vi "Dashboard Main.vi"() -> ()   [LabVIEW 2015]
uses:
  <vilib>/Utility/miscctls.llb/LVRowAndColumnTypeDef.ctl
  <vilib>/event_ctls.llb/eventvkey.ctl
  <vilib>/Rock Robotics/WPI/Dashboard/WPI_DashboardLogging Global.vi
  <vilib>/Rock Robotics/Network Tables/NT Read Numeric Array.vi
  <vilib>/Rock Robotics/Network Tables/SD Write Number.vi
  <vilib>/Rock Robotics/Network Tables/NT Write Boolean.vi
  <vilib>/Rock Robotics/Network Tables/NT Read Boolean.vi
  <vilib>/Utility/config.llb/Write Key (String).vi
  <vilib>/Utility/config.llb/Write Key (I32).vi
  <vilib>/Utility/config.llb/NI_LVConfig.lvlib
panel:
  in  "Vision 2":u16(ring)=3 items=["IP Camera"=3]
  out "Camera Image 2":T1(plugin-control)
  in  "TCP":refnum<k5>
  in  "Rec Mode":enum32{"Stop", "Record", "Playback"}(radio)
  in  "Vision":u16(ring)=1 items=["USB Cam"=1]
  out "Camera IP":string
  out "Image Message":string="Timeout in Camera Communications"
  in  "Dashboard Tab":T2(tab)
  in  "Camera Settings":T3={"Frame Rate"=30, "Compression"=30, "Size"=1} {"Frame Rate" scale=1.0..30.0; "Size" items=["640x480", "320x240", "160x120"]}
  out "Mode":T4(ring)=enum."Auto Disabled"
  in  "DB Camera Config":bool
  out "fps":dbl format="%#.1g"
  out "Mbps":dbl format="%#.1g"
  out "Mbps LED":bool
  in  "Autonomous Select":T5(ring)
  in  "Top Speed":dbl=1300.0 min=0.0 max=2.0 step=0.01
  in  "Intake Speed":dbl=1.0 min=0.0 max=1.0 step=0.01
  in  "Bottom Speed":dbl=2100.0 min=0.0 max=2.0 step=0.01
  in  "First  Drive":dbl=180.0 min=0.0 max=2.0 step=0.01
  in  "First Turn":dbl=39.0 min=0.0 max=1.0 step=0.01
  in  "Second Turn":dbl min=0.0 max=1.0 step=0.01
  in  "Second Drive":dbl=72.0 min=0.0 max=2.0 step=0.01
  in  "PID Control":bool=TRUE
  out "Bottom Encoder Velocity":dbl(knob) scale=0.0..3000.0
  out "Top Wop":bool
  out "Bottom Floop":bool
  out "Override":bool
  out "SHOOT!":bool
  in  "Auto Shoot":bool=TRUE
  in  "Release Speed":dbl=2090.0
  out "Line  Break":bool
  out "x":dbl
  out "y":dbl
  in  "Release Time":dbl=2090.0
  out "angle":dbl
  out "scale":dbl
  in  "DB/String 9":string
  in  "DB/String 8":string
  in  "DB/String 7":string
  in  "DB/String 6":string
  in  "DB/String 5":string
  in  "DB/String 4":string
  in  "DB/String 3":string
  in  "DB/String 2":string
  in  "DB/String 1":string
  in  "DB/String 0":string
  in  "DB/Slider 0":dbl(slide) scale=0.0..5.0
  in  "DB/Slider 1":dbl(slide) scale=0.0..5.0
  in  "DB/Slider 2":dbl(slide) scale=0.0..5.0
  in  "DB/Slider 3":dbl(slide) scale=0.0..5.0
  out "DB/LED 3":bool
  out "DB/LED 2":bool
  out "DB/LED 1":bool
  out "DB/LED 0":bool
  in  "DB/Button 3":bool
  in  "DB/Button 2":bool
  in  "DB/Button 1":bool
  in  "DB/Button 0":bool caption="New Name"
  out "Mbps 2":dbl format="%#.1g"
  in  "Camera Settings 2":T3={"Frame Rate"=30, "Compression"=30, "Size"=1} {"Frame Rate" scale=1.0..30.0; "Size" items=["640x480", "320x240", "160x120"]}
  out "fps 2":dbl format="%#.1g"
  in  "Rec Mode 2":enum32{"Stop", "Record", "Playback"}(radio)
  in  "Top P":dbl=3.0 min=0.0 max=2.0 step=0.01
  in  "Top I":dbl=0.01 min=0.0 max=1.0 step=0.01
  in  "Top D":dbl=7.0 min=0.0 max=2.0 step=0.01
  in  "Bottom P":dbl=3.0 min=0.0 max=2.0 step=0.01
  in  "Bottom I":dbl=0.01 min=0.0 max=1.0 step=0.01
  in  "Bottom D":dbl=12.0 min=0.0 max=2.0 step=0.01
  out "Gyro":dbl(knob) scale=0.0..360.0
  out "Top Encoder Velocity":dbl(knob) scale=0.0..3000.0
  in  "Gyro Reset":bool
  in  "Right Drive Reset":bool
  in  "Left Drive Reset":bool
  out "Left Drive Encoder":dbl
  out "Right Drive Encoder":dbl
  in  "X Offset":dbl min=0.0 max=1.0 step=0.01
  in  "Y Offset":dbl min=0.0 max=1.0 step=0.01
  in  "Angle Offset":dbl min=0.0 max=1.0 step=0.01
  in  "Scale Offset":dbl min=0.0 max=1.0 step=0.01
  in  "Test Slider":dbl(slide) scale=0.0..100.0 scale format="%#_3g"
  in  "On/Off":bool caption="Solenoid"
  in  "Test Name":u16(ring) items=["Select the test to run..."]
  in  "Test Tree":string(tree)
  in  "Motor":cluster{"Value":dbl, "Enable":bool} {"Value" scale=-1.0..1.0 scale format="%#_3g"}
  out "Progress":T6 {"Test Progress" scale=0.0..100.0}
  in  "Rev/Fwd":cluster{"Forward":bool, "Reverse":bool}
  in  "Test Ring":u16(ring) items=["Monochrome", "Color"]
  out "Cmd Status":string
  in  "Execute Command":bool
  in  "Command Params":string[][](table)
  in  "Command Selection":i32(listbox)
  in  "Select Auto":string(combo)
  out "JS2 Z":dbl(slide) scale=-1.0..1.0 scale format="%#_2e"
  out "JS2 Graph":cluster{"X":dbl, "Y":dbl}[](graph)
  out "JS2 Buttons":T7
  out "JS1 Z":dbl(slide) scale=-1.0..1.0 scale format="%#_2e"
  out "JS1 Graph":cluster{"X":dbl, "Y":dbl}[](graph)
  out "JS1 Buttons":T7
  in  "CheckList":i32(listbox)
  out "Tree":string(tree)
  out "Camera Image":T1(plugin-control)
  out "Background":bool
  # "This tab is a great place for autonomous settings and robot-specific values.\nPlace controls and indicators inside this tab and match name to\nDashboard Variables on robot. You can also delete this comment."
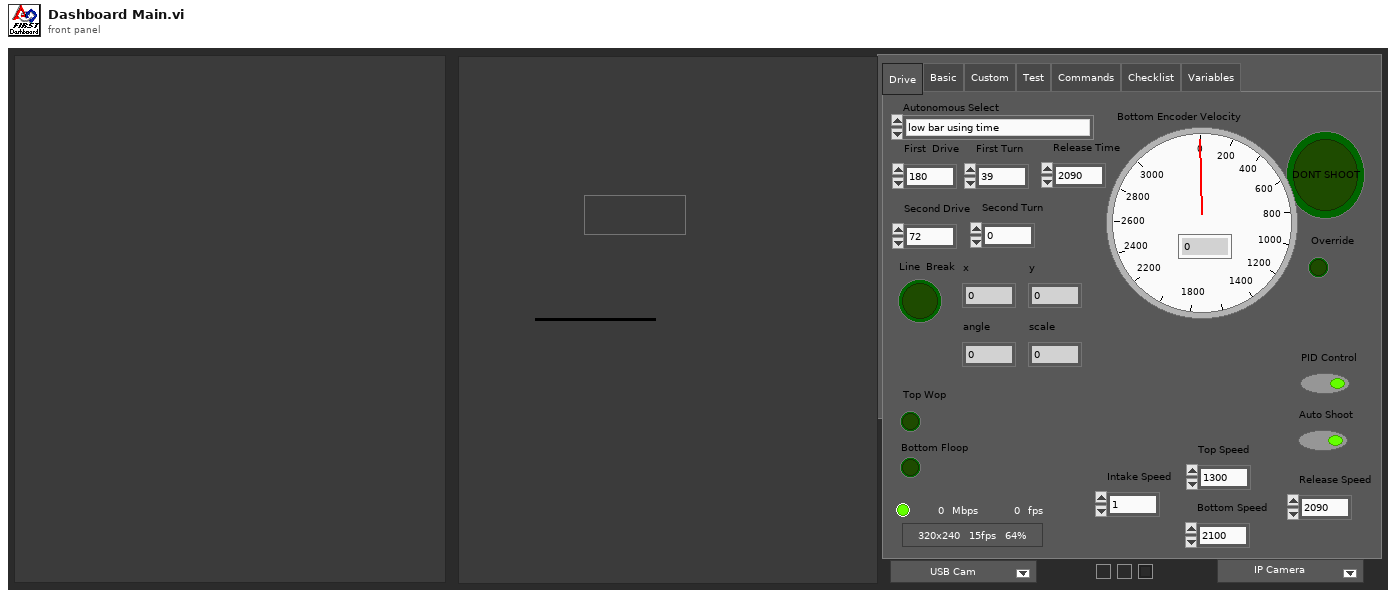
[diagram p1: front panel]
types:
  T1 = typedef "IMAQ Image.ctl" = refnum<image>
  T2 = enum32{"Drive", "Basic", "Custom", "Test", "Commands", "Checklist", "Variables"}
  T3 = cluster{"Frame Rate":i32, "Compression":i32, "Size":u16}
  T4 = enum8{"Tele-Op Disabled", "Tele-Op Enabled", "Auto Disabled", "Auto Enabled", "Test Disabled", "Test Enabled", "Disconnected", "No Code", "E-Stop"}
  T5 = enum16{"low bar using time", "low goal from low bar", "high goal from low bar", "rough terrain", "STRAIGHT FORWARD", "Do nothing", "low bar with encoder", "SHIMMY AUTO", "just touching", "Portcullis", "Cheval", "Vision 3rd Position", "Vision Test", "Bennett's Vision Code"}
  T6 = cluster{"Test Progress":u8, "Test Progress Text":string}
  T7 = cluster{bool, bool, bool, bool, bool, bool, bool, bool, bool, bool, bool, bool}
  T8 = typedef "Image Type" = u32
  T9 = cluster{"IDs":cluster{"RPC field ID":u16, "Unique ID":u16}, "String":string}
  T10 = enum32{"Drive", "Basic", "Custom", "Test", "Checklist", "Variables"}
  T11 = cluster{"Camera Image":refnum<vi>, "Dashboard Tab":refnum<vi>, "Background":refnum<vi>, "Vision":refnum<vi>, "Rec Mode":refnum<vi>, "Test Slider":refnum<vi>, "On/Off ":refnum<vi>, "Test Ring":refnum<vi>, "Rev/Fwd":refnum<vi>, "Test Name":refnum<vi>, "Motor":refnum<vi>, "Progress":refnum<vi>, "CheckList":refnum<vi>, "Tree":refnum<vi>, "Test Tree":refnum<vi>, "Command Params":refnum<vi>, "Command Selection":refnum<vi>, "Execute Command":refnum<vi>, "Cmd Status":refnum<vi>}
  T12 = cluster{"Position":cluster{"x":sgl, "y":sgl}, "Angle":sgl, "Scale":sgl, "Score":sgl, "Bounding Box":cluster{"x":sgl, "y":sgl}[]}[]
  T13 = cluster{"Position":cluster{"x":sgl, "y":sgl}, "Angle":sgl, "Scale":sgl, "Score":sgl, "Bounding Box":cluster{"x":sgl, "y":sgl}[]}
  T14 = typedef "NI_LVConfig.lvlib/Config Data RefNum.ctl" = refnum<k1>
  T15 = cluster{"Error Strings":string, "Disable Counts":cluster{u16, u16}, "Rail Faults":cluster{u16, u16, u16}, "Robot IP":string, "DB Mode":u8, "Event Info":cluster{"Name":string, "Type":u8, "Number":u16, "Replay":u8}, "Camera Addr":string}
  T16 = cluster{"Storage":cluster{"Disk Free":u64, "RAM Block":u32, "RAM free":u32}, "CPU Utilization":cluster{"CPU % ISR":sgl, "CPU % Time Crit":sgl, "CPU % Timed Str":sgl, "CPU % High":sgl, "CPU % Above":sgl, "CPU % Normal":sgl, "CPU % Low":sgl}, "CAN":cluster{"% Bus Utilization":sgl, "Bus Off Cnt":u32, "TX_FIFO Full Cnt":u32, "Receive Error Cnt":u8, "Transmit Error Cnt":u8}, "HID":cluster{"HID Outputs":u32, "Rumble Low":u16, "Rumble High":u16}[]}
  T17 = cluster{"Status bits":cluster{"Test Mode":bool, "Autonomous":bool, "Enabled":bool, "Code Start":bool, "Brownout":bool, "Reserved 2":bool, "Reserved 3":bool, "E-Stop":bool}, "Code Trace":cluster{"Disabled":bool, "TeleOp":bool, "Auto":bool, "Test":bool}, "Controller Type":enum16{"unknown", "cRIO", "roboRio"}, "Code?":enum16{"unknown", "noCode", "code"}, "Battery V":dbl}
  T18 = cluster{"Control Bits":cluster{"TestMode":bool, "Autonomous":bool, "Enabled":bool, "FMS Present":bool, bool, bool, bool, "E-Stop":bool}, "Team Station ":u8, "Countdown":sgl, "Joystick Values":cluster{"Axes":dbl[], "Buttons":bool[], "POVs":i16[]}[]}
  T19 = cluster{"Axes":dbl[], "Buttons":bool[], "POVs":i16[]}[]
  T20 = cluster{"Axes":dbl[], "Buttons":bool[], "POVs":i16[]}
  T21 = cluster{"Buttons[0]":bool, "Buttons[1]":bool, "Buttons[2]":bool, "Buttons[3]":bool, "Buttons[4]":bool, "Buttons[5]":bool, "Buttons[6]":bool, "Buttons[7]":bool, "Buttons[8]":bool, "Buttons[9]":bool, "Buttons[10]":bool, "Buttons[11]":bool}
  T22 = cluster{"Operation":enum16{"Update", "Clear"}, "Color Box":u32}[]
  T23 = typedef "eventvkey.ctl" = enum16{"ASCII", "Enter", "Return", "Shift", "Ctrl", "Alt", "Cmd", "Opt", "Caps", "NumLock", "Clear", "Break", "Up", "Down", "Left", "Right", "Insert", "Delete", "Home", "End", "PageUp", "PageDown", "Escape", "Help", "Pause", "ScrollLock", "F1", "F2", "F3", "F4", "F5", "F6", "F7", "F8", "F9", "F10", "F11", "F12", "F13", "F14", "F15", "F16", "F17", "F18", "F19", "F20", "F21", "F22", "F23", "F24", "Play", "VolumeUp", "VolumeDown", "Mute", "Two Byte Char"}
  T24 = cluster{"Image Size":bool, "Image Type":bool, "Pixel Value":bool, "ROI Information":bool, "Zoom Factor":bool}
  T25 = enum8{"Enabled", "Disabled", "Disabled and Grayed Out"}
  T26 = cluster{"Operation":enum16{"Update", "Clear"}, "Color Box":u32}
  T27 = typedef "LVRowAndColumnTypeDef.ctl" = cluster{"Row":i32, "Column":i32}
  T28 = cluster{"Shift":bool, "Ctrl":bool, "Alt":bool, "Cmd":bool, "Opt":bool}
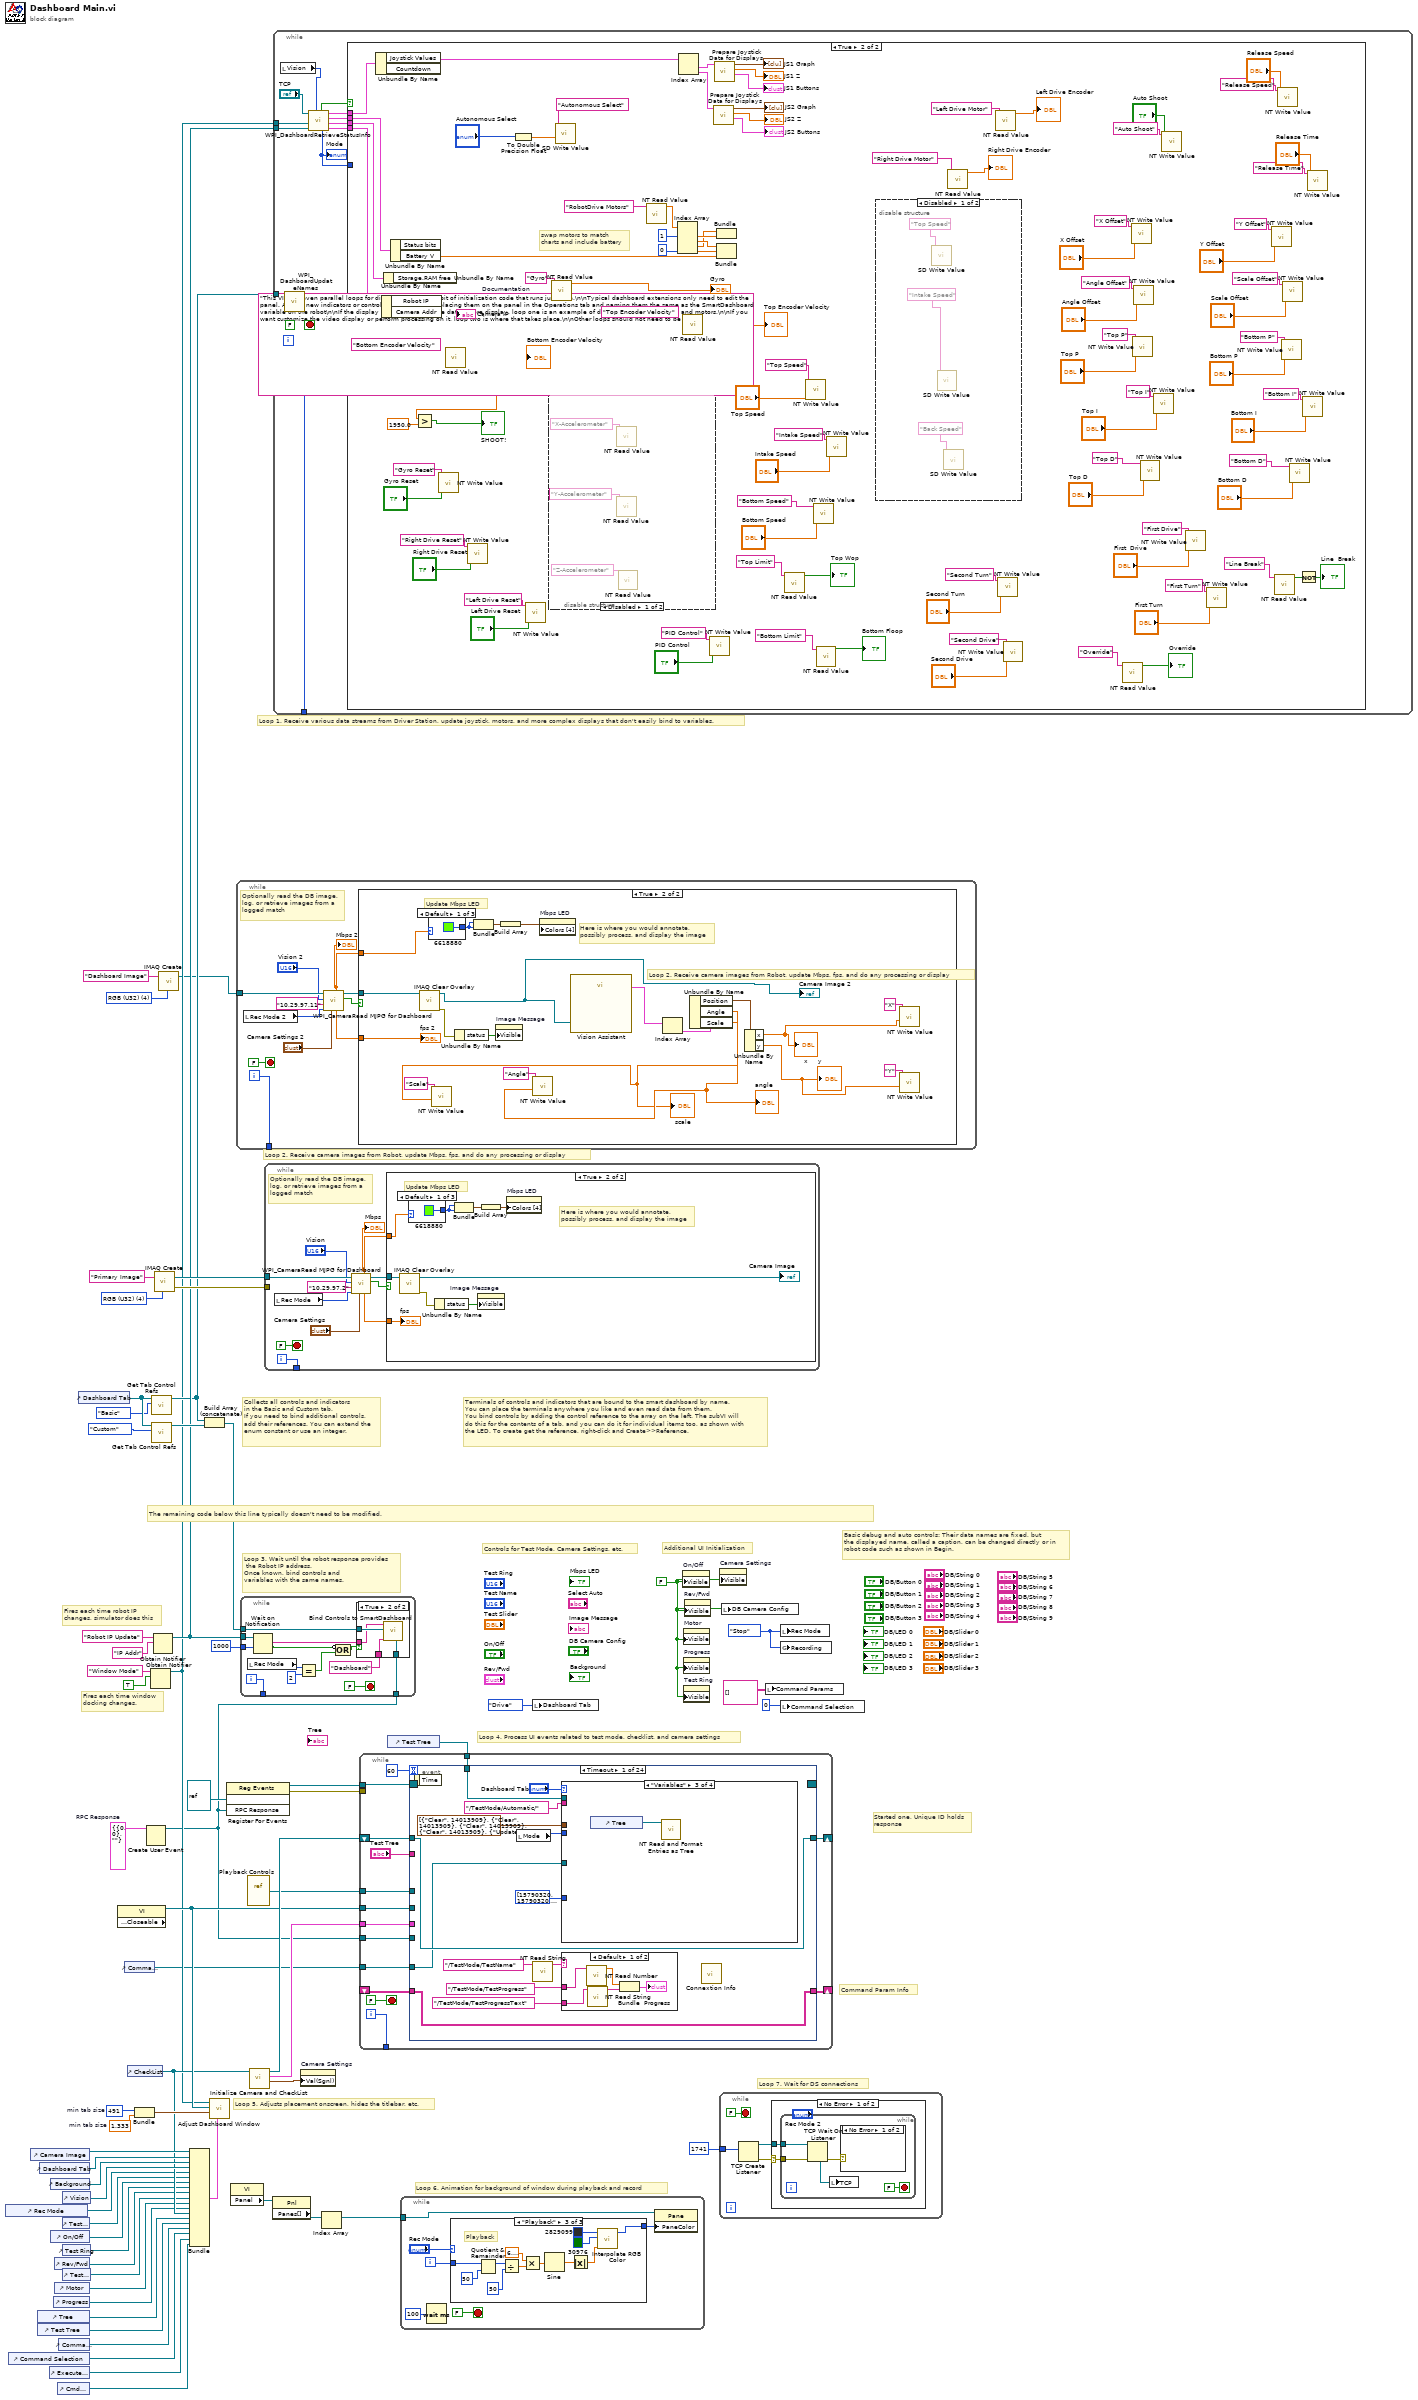
[diagram p0: block diagram]
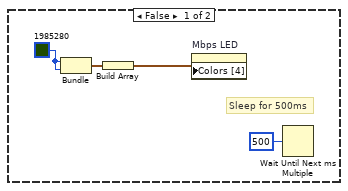
[diagram p2: hidden frame]
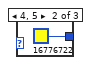
[diagram p3: hidden frame]
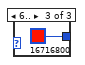
[diagram p4: hidden frame]
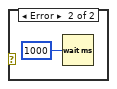
[diagram p5: hidden frame]
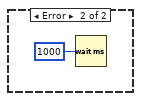
[diagram p6: hidden frame]
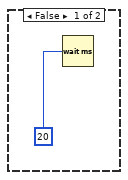
[diagram p7: hidden frame]
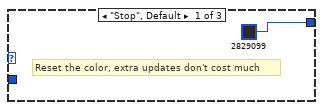
[diagram p10: hidden frame]
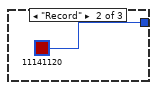
[diagram p11: hidden frame]
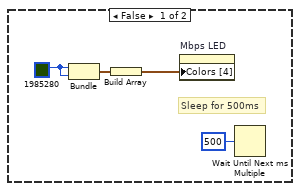
[diagram p13: hidden frame]
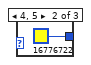
[diagram p14: hidden frame]
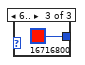
[diagram p15: hidden frame]
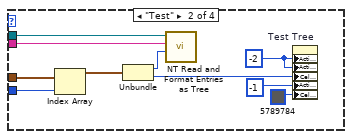
[diagram p17: hidden frame]
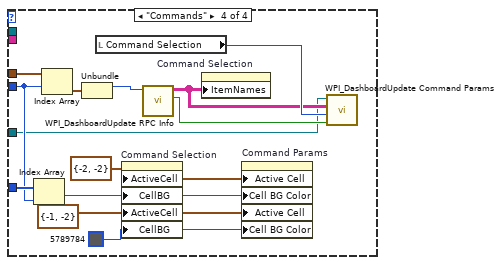
[diagram p18: hidden frame]
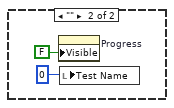
[diagram p19: hidden frame]
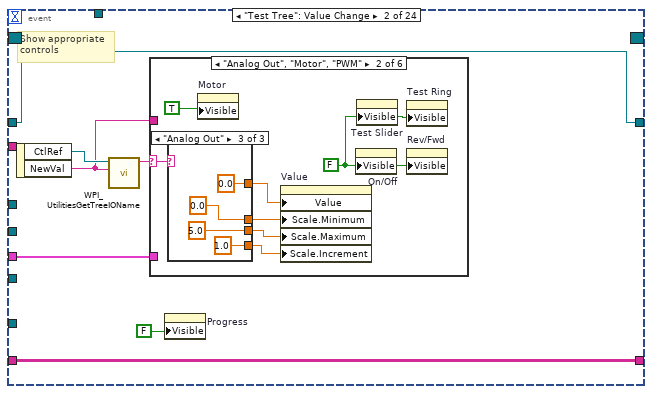
[diagram p20: hidden frame]
diagram:
  w2 = T8 4 items=["Grayscale (U8)", "Grayscale (I16)", "Grayscale (SGL)", "Complex (CSG)", "RGB (U32)", "HSL (U32)", "RGB (U64)"] ("Image Type")
  w10 = T9 {"IDs"={"RPC field ID"=0, "Unique ID"=0}, "String"=""}  # RPC Response
  w36 = 491  # min tab size
  w35 = 1.333  # min tab size
  w44 = enum32{"Stop", "Record", "Playback"}."Stop" ("Rec Mode")
  w18 = FALSE ("Visible")
  (unwired) "This VI has seven parallel loops for different tasks and a bit of initialization code that runs just once.\n\nTypical dashboard extensions only need to edit the panel. Adding new indicators or controls simply involves placing them on the panel in the Operations tab and naming them the same as the SmartDashboard variable on the robot\n\nIf the display needs to process the data before display, loop one is an example of doing that for the joysticks and motors.\n\nIf you want customize the video display or perform processing on it, loop two is where that takes place.\n\nOther loops should not need to be modified. They are pretty standard, and document the task they perform."  # Documentation
  w64 = T8 4 items=["Grayscale (U8)", "Grayscale (I16)", "Grayscale (SGL)", "Complex (CSG)", "RGB (U32)", "HSL (U32)", "RGB (U64)"] ("Image Type")
  # "Loop 2. Receive camera images from Robot, update Mbps, fps, and do any processing or display"
  # "Command Param Info"
  # "Started one, Unique ID holds\nresponse"
  # "Loop 7. Wait for DS connections"
  # "Basic debug and auto controls: Their data names are fixed, but\nthe displayed name, called a caption, can be changed directly or in\nrobot code such as shown in Begin."
  # "Controls for Test Mode, Camera Settings, etc."
  # "Additional UI Initialization"
  # "Loop 6. Animation for background of window during playback and record"
  # "Fires each time robot IP\nchanges, simulator does this"
  # "Fires each time window\ndocking changes."
  # "Collects all controls and indicators\nin the Basic and Custom tab.\nIf you need to bind additional controls,\nadd their references. You can extend the\nenum constant or use an integer."
  # "The remaining code below this line typically doesn't need to be modified."
  # "Loop 4. Process UI events related to test mode, checklist, and camera settings"
  # "Terminals of controls and indicators that are bound to the smart dashboard by name.\nYou can place the terminals anywhere you like and even read data from them.\nYou bind controls by adding the control reference to the array on the left. The subVI will\ndo this for the contents of a tab, and you can do it for individual items too, as shown with\nthe LED. To create get the reference, right-click and Create>>Reference."
  # "Loop 3. Wait until the robot response provides\n the Robot IP address.\nOnce known, bind controls and\nvariables with the same names."
  # "Loop 5. Adjusts placement onscreen, hides the titlebar, etc."
  # "Loop 1. Receive various data streams from Driver Station, update joystick, motors, and more complex displays that don't easily bind to variables."
  # "Loop 2. Receive camera images from Robot, update Mbps, fps, and do any processing or display"
  n1 = control-ref of="Rec Mode"() -> (w24:refnum<vi>)
  n2 = control-ref of="Command Selection"() -> (w9:refnum<vi>)
  n3 = control-ref of="Camera Image"() -> (w39:refnum<vi>)
  n4 = control-ref of="Tree"() -> (w28:refnum<vi>)
  n5 = control-ref of="Test Tree"() -> (w27:refnum<vi>)
  n6 = control-ref of="Dashboard Tab"() -> (w38:refnum<vi>)
  n7 = control-ref of="Execute Command"() -> (w11:refnum<vi>)
  n8 = control-ref of="Background"() -> (w33:refnum<vi>)
  n9 = control-ref of="On/Off"() -> (w22:refnum<vi>)
  n10 = control-ref of="Progress"() -> (w19:refnum<vi>)
  n11 = control-ref of="Rev/Fwd"() -> (w20:refnum<vi>)
  n12 = control-ref of="Motor"() -> (w25:refnum<vi>)
  n13 = control-ref of="Cmd Status"() -> (w5:refnum<vi>)
  n14 = control-ref of="Command Params"() -> (w12:refnum<vi>)
  n15 = control-ref of="Test Slider"() -> (w23:refnum<vi>)
  n16 = control-ref of="Vision"() -> (w37:refnum<vi>)
  n17 = control-ref of="Test Ring"() -> (w21:refnum<vi>)
  n18 = control-ref of="Test Name"() -> (w26:refnum<vi>)
  n19 = control-ref of="Dashboard Tab"() -> (w42:refnum<vi>)
  n20 = property class="VI" props=["Front Panel.Closeable"]() -> (reference out=w43:refnum<vi>)  [unwired: 2 in, 2 out]
  n21 = control-ref of="Command Params"() -> (w4:refnum<vi>)
  n22 = control-ref of="CheckList"() -> (w29:refnum<vi>)
  n23 = Bundle("min tab size"=w36, "min tab size"=w35) -> (w34:cluster{"min tab size":i32, "min tab size":dbl})  [unwired: 1 in]
  n24 = Create User Event(user event datatype=w10) -> (user event=w6:refnum<user-event>)  [unwired: 1 in, 1 out]
  n25 = Obtain Notifier(name (unnamed)="Window Mode", notification data type=TRUE) -> (notifier out=w15:refnum<notifier>)  [unwired: 2 in, 2 out]
  n26 = call <vilib>:"Get Tab Control Refs.vi"("Page Index"=T10."Basic" ("Dashboard Tab"), "TabControl in"=w42) -> ("ControlsOnPage"=w16:refnum<vi>[])  [unwired: 9 in]
  n27 = call <vilib>:"Get Tab Control Refs.vi"("Page Index"=T10."Custom" ("Dashboard Tab"), "TabControl in"=w42) -> ("ControlsOnPage"=w41:refnum<vi>[])  [unwired: 9 in]
  n28 = Obtain Notifier(name (unnamed)="Robot IP Update", notification data type="IP Addr" ("name (unnamed)")) -> (notifier out=w17:refnum<notifier>)  [unwired: 2 in, 2 out]
  n29 = call "IMAQ Create"("Image Name"="Primary Image", "Image Type"=w64) -> ("New Image"=w62:T1, "error out"=w61:errorcluster)  [unwired: 2 in, 1 out]
  n30 = call "IMAQ Create"("Image Name"="Dashboard Image", "Image Type"=w2) -> ("New Image"=w1:T1)  [unwired: 2 in, 2 out]
  n31 = Bundle("Camera Image"=w39, "Dashboard Tab"=w38, "Background"=w33, "Vision"=w37, "Rec Mode"=w24, "Test Slider"=w23, "On/Off"=w22, "Test Ring"=w21, "Rev/Fwd"=w20, "Test Name"=w26, "Motor"=w25, "Progress"=w19, "CheckList"=w29, "Tree"=w28, "Test Tree"=w27, "Command Params"=w12, "Command Selection"=w9, "Execute Command"=w11, "Cmd Status"=w5) -> (w30:T11)  [unwired: 1 in]
  n32 = Build Array (concatenate)(w16, w41) -> (w40:refnum<vi>[])
  n33 = call "Adjust Dashboard Window.vi"("Sizing Refnums"=w30, "Size Constraints"=w34, "VI"=w43, "WIn Mode"=w15) -> ()  [unwired: 8 in]
  n34 = register-events(refnum<vi> refnum, w6) -> (reference out=w48:refnum<event-registration>, error out=w47:errorcluster)  [unwired: 2 in]
  n35 = property class="VI"() -> ("Panel"=w51:refnum<vi>)  [unwired: 2 in, 2 out]
  n36 = while {
    tunnel: w1 -> [w73]
    tunnel: [w74] -> _
    i -> [w74]
    stop <- FALSE stop-if-true
    # "Optionally read the DB image,\nlog, or retrieve images from a\nlogged match"
    n37 = local read "Rec Mode 2"() -> (w68:enum32{"Stop", "Record", "Playback"})
    n38 = call <vilib>:"WPI_CameraRead MJPG for Dashboard.vi"("Camera Settings"="Camera Settings 2", "Rec Mode"=w68, "Camera IP"="10.29.97.11", "Camera Mode"="Vision 2", "Refnum in"=w73) -> ("Active"=w71:bool, "Refnum out"=w72:T1, "FPS"=w70:dbl, "Bandwidth (Mbps)"=w66:dbl)  [unwired: 3 in]
    "Mbps 2" <- w66
    n39 = case shown="True" w71 {
      tunnel: w72 -> [_ w96]
      tunnel: w66 -> [_ w95]
      tunnel: w70 -> [_ w94]
      frame False {
        w77 = u32 1985280 ("Color Box")
        # "Sleep for 500ms"
        n40 = Bundle("Color Box"=w77, "Color Box"=w77) -> (w78:cluster{"Color Box":u32, "Color Box":u32})  [unwired: 1 out]
        n41 = Build Array(w78) -> (w76:cluster{"Color Box":u32, "Color Box":u32}[])
        n42 = property on="Mbps LED" class="Bool (strict)"("Colors [4]"=w76) -> ()  [unwired: 2 in, 2 out]
        n43 = Wait Until Next ms Multiple(millisecond multiple=u32 500) -> ()  [unwired: 1 out]
      }
      frame True {
        # "Here is where you would annotate,\npossibly process, and display the image"
        # "Update Mbps LED"
        n44 = call "IMAQ Clear Overlay"("Image"=w96) -> ("error out"=w99:errorcluster, "Image Out"=w80:T1)  [unwired: 2 in, 7 out]
        "Camera Image 2" <- w80
        n45 = case shown="Default" w95 {
          tunnel: [u32 6618880 ("Color Box") u32 16776722 ("Color Box") u32 16716800 ("Color Box")] -> w97
          frame Default {
          }
          frame 4, 5 {
          }
          frame 6.. {
          }
        }
        n46 = Unbundle By Name(w99) -> ("status"=w92:bool)
        n47 = Bundle("Color Box"=w97, "Color Box"=w97) -> (w98:cluster{"Color Box":u32, "Color Box":u32})  [unwired: 1 out]
        n48 = property on="Image Message" class="Str"("Visible"=w92) -> ()  [unwired: 2 in, 2 out]
        n49 = Build Array(w98) -> (w93:cluster{"Color Box":u32, "Color Box":u32}[])
        n50 = property on="Mbps LED" class="Bool (strict)"("Colors [4]"=w93) -> ()  [unwired: 2 in, 2 out]
        n51 = call "Vision Assistant"("Image In"=w80) -> ("Calibrated Matches (Pattern Matching 1)"=w89:T12)  [unwired: 22 in, 4 out]
        n52 = Index Array(array=w89) -> (element=w91:T13)  [unwired: 1 in]
        n53 = Unbundle By Name(w91) -> ("Position"=w90:cluster{"x":sgl, "y":sgl}, "Angle"=w82:sgl, "Scale"=w81:sgl)
        "angle" <- w82
        "scale" <- w81
        n54 = call-poly <vilib>:"NT Write Value.vi"("Numeric"=w81, "Name"="Scale") -> ()  [unwired: 9 in, 1 out]
        n55 = call-poly <vilib>:"NT Write Value.vi"("Numeric"=w82, "Name"="Angle") -> ()  [unwired: 9 in, 1 out]
        n56 = Unbundle By Name(w90) -> ("x"=w87:sgl, "y"=w85:sgl)
        "x" <- w87
        "y" <- w85
        n57 = call-poly <vilib>:"NT Write Value.vi"("Numeric"=w87, "Name"="X") -> ()  [unwired: 9 in, 1 out]
        n58 = call-poly <vilib>:"NT Write Value.vi"("Numeric"=w85, "Name"="Y") -> ()  [unwired: 9 in, 1 out]
        "fps 2" <- w94
      }
    }
  }
  n59 = while {
    tunnel: w40 -> [w115]
    tunnel: w17 -> [w113]
    tunnel: [w111] -> _
    tunnel: u32 1000 ("milliseconds to wait") -> [w110]
    tunnel: w6 -> [w103]
    i -> [w111]
    stop <- FALSE stop-if-true
    n60 = local read "Rec Mode"() -> (w106:enum32{"Stop", "Record", "Playback"})
    n61 = Wait on Notification(notifier=w113, timeout in ms (-1)=w110) -> (notification=w112:string, timed out?=w108:bool)  [unwired: 2 in, 2 out]
    n62 = Equal?(x=w106, y=u16 2 ("Rec Mode")) -> (x = y?=w107:bool)
    n63 = Compound Arithmetic op=OR(invert w108, w107) -> (w109:bool)
    n64 = case shown="True" w109 {
      tunnel: w115 -> [_ w119]
      tunnel: w112 -> [_ w118]
      tunnel: "Dashboard" -> [_ w117]
      tunnel: w103 -> [_ w116]
      frame False {
      }
      frame True {
        n65 = call <vilib>:"Bind Controls to SmartDashboard.vi"("RPC ref"=w116, "Client Name"=w117, "Bound Control Refs"=w119, "Server IP Address"=w118) -> ()  [unwired: 8 in]
      }
    }
  }
  n66 = vi-ref "Playback Controls.vi"() -> (w49:refnum<vi>)
  n67 = call "Initialize Camera and CheckList.vi"("ListBox in"=w29) -> ("Cluster"=w55:cluster{"value":i32, "value":i32, "index":i32}, "Array"=w56:cluster{string[]}[], "File Refnum"=w54:T14)  [unwired: 8 in]
  n68 = while {
    tunnel: w62 -> [w128]
    tunnel: w61 -> [_]
    tunnel: [w129] -> _
    i -> [w129]
    stop <- FALSE stop-if-true
    # "Optionally read the DB image,\nlog, or retrieve images from a\nlogged match"
    n69 = local read "Rec Mode"() -> (w123:enum32{"Stop", "Record", "Playback"})
    n70 = call <vilib>:"WPI_CameraRead MJPG for Dashboard.vi"("Camera Settings"="Camera Settings", "Rec Mode"=w123, "Camera IP"="10.29.97.2", "Camera Mode"="Vision", "Refnum in"=w128) -> ("Active"=w126:bool, "Refnum out"=w127:T1, "FPS"=w125:dbl, "Bandwidth (Mbps)"=w121:dbl)  [unwired: 3 in]
    "Mbps" <- w121
    n71 = case shown="True" w126 {
      tunnel: w127 -> [_ w138]
      tunnel: w121 -> [_ w137]
      tunnel: w125 -> [_ w135]
      frame False {
        w131 = u32 1985280 ("Color Box")
        # "Sleep for 500ms"
        n72 = Bundle("Color Box"=w131, "Color Box"=w131) -> (w133:cluster{"Color Box":u32, "Color Box":u32})  [unwired: 1 out]
        n73 = Build Array(w133) -> (w132:cluster{"Color Box":u32, "Color Box":u32}[])
        n74 = property on="Mbps LED" class="Bool (strict)"("Colors [4]"=w132) -> ()  [unwired: 2 in, 2 out]
        n75 = Wait Until Next ms Multiple(millisecond multiple=u32 500) -> ()  [unwired: 1 out]
      }
      frame True {
        # "Here is where you would annotate,\npossibly process, and display the image"
        # "Update Mbps LED"
        n76 = call "IMAQ Clear Overlay"("Image"=w138) -> ("error out"=w142:errorcluster, "Image Out"=→"Camera Image":T1)  [unwired: 2 in, 7 out]
        n77 = case shown="Default" w137 {
          tunnel: [u32 6618880 ("Color Box") u32 16776722 ("Color Box") u32 16716800 ("Color Box")] -> w139
          frame Default {
          }
          frame 4, 5 {
          }
          frame 6.. {
          }
        }
        n78 = Unbundle By Name(w142) -> ("status"=w143:bool)
        n79 = Bundle("Color Box"=w139, "Color Box"=w139) -> (w141:cluster{"Color Box":u32, "Color Box":u32})  [unwired: 1 out]
        n80 = property on="Image Message" class="Str"("Visible"=w143) -> ()  [unwired: 2 in, 2 out]
        n81 = Build Array(w141) -> (w140:cluster{"Color Box":u32, "Color Box":u32}[])
        n82 = property on="Mbps LED" class="Bool (strict)"("Colors [4]"=w140) -> ()  [unwired: 2 in, 2 out]
        "fps" <- w135
      }
    }
  }
  n83 = property class="Pnl"(reference=w51) -> ("Panes[]"=w52:refnum<vi>[])  [unwired: 1 in, 2 out]
  n84 = while {
    tunnel: [w158] -> _
    tunnel: w17 -> [w152]
    tunnel: w16 -> [w151]
    tunnel: w15 -> [w147]
    i -> [w158]
    stop <- FALSE stop-if-true
    n85 = local read "Vision"() -> (w149:u16)
    n86 = call <vilib>:"WPI_DashboardUpdateNames.vi"("Controls on Tab"=w151) -> ()  [unwired: 11 in]
    n87 = call <vilib>:"WPI_DashboardRetrieveStatusInfo.vi"("Vision"=w149, "Binding Refnum"=w152, "Window Mode Notifier"=w147, "TCP Cnx"="TCP") -> ("Power and Errors"=w153:T15, "Robot Metrics"=w156:T16, "Status Info"=w157:T17, "Control Info"=w154:T18, "Robot Mode"=w150:T4, "Process?"=w155:bool)  [unwired: 2 in]
    "Mode" <- w150
    n88 = case shown="True" w155 {
      tunnel: w157 -> [_ w255]
      tunnel: w156 -> [_ w254]
      tunnel: w154 -> [_ w253]
      tunnel: w153 -> [_ w252]
      tunnel: w150 -> [_ _]
      frame False {
        n89 = Wait (ms)(milliseconds to wait=u32 20) -> ()  [unwired: 1 out]
      }
      frame True {
        # "swap motors to match\ncharts and include battery"
        n90 = Unbundle By Name(w253) -> ("Joystick Values"=w244:T19)  [unwired: 1 out]
        n91 = Unbundle By Name(w252) -> ("Camera Addr"=→"Camera IP":string)  [unwired: 1 out]
        n92 = Unbundle By Name(w254) -> ()  [unwired: 1 out]
        n93 = Unbundle By Name(w255) -> ("Battery V"=w245:dbl)  [unwired: 1 out]
        n94 = call-poly <vilib>:"NT Write Value.vi"("Boolean"="Gyro Reset", "Name"="Gyro Reset") -> ()  [unwired: 9 in, 1 out]
        n95 = call-poly <vilib>:"NT Read Value.vi"("Name"="Bottom Encoder Velocity") -> ("Numeric"=w175:dbl)  [unwired: 9 in, 1 out]
        "Bottom Encoder Velocity" <- w175
        n96 = Greater?(x=w175, y=1950.0) -> (0:→"SHOOT!":bool)
        n97 = call-poly <vilib>:"NT Write Value.vi"("Boolean"="Right Drive Reset", "Name"="Right Drive Reset") -> ()  [unwired: 9 in, 1 out]
        n98 = To Double Precision Float(number="Autonomous Select") -> (double precision float=w230:dbl)
        n99 = call-poly <vilib>:"NT Write Value.vi"("Boolean"="Left Drive Reset", "Name"="Left Drive Reset") -> ()  [unwired: 9 in, 1 out]
        n100 = disable-structure shown="Disabled" {
          frame Disabled {
            n101 = call-poly <vilib>:"NT Read Value.vi"("Name"="Y-Accelerometer") -> ("Numeric"=w266:dbl)  [unwired: 9 in, 1 out]
            n102 = call-poly <vilib>:"NT Read Value.vi"("Name"="X-Accelerometer") -> ("Numeric"=w265:dbl)  [unwired: 9 in, 1 out]
            n103 = call-poly <vilib>:"NT Read Value.vi"("Name"="Z-Accelerometer") -> ("Numeric"=w263:dbl)  [unwired: 9 in, 1 out]
          }
          frame Enabled {
          }
        }
        n104 = call-poly <vilib>:"NT Read Value.vi"("Name"="Gyro") -> ("Numeric"=→"Gyro":dbl)  [unwired: 9 in, 1 out]
        n105 = call-poly <vilib>:"SD Write Value.vi"("Numeric"=w230, "Name"="Autonomous Select") -> ()  [unwired: 8 in, 2 out]
        n106 = call-poly <vilib>:"NT Read Value.vi"("Name"="RobotDrive Motors") -> ("Numeric Array"=w233:dbl[])  [unwired: 9 in, 1 out]
        n107 = Index Array(array=w233, index #1=1, index #4=0) -> (element #1=w247:dbl, element #2=w248:dbl, element #3=w246:dbl, element #4=w251:dbl)  [unwired: 2 in]
        n108 = Index Array(array=w244) -> (element #1=w243:T20, element #2=w238:T20)  [unwired: 2 in]
        n109 = call-poly <vilib>:"NT Read Value.vi"("Name"="Top Encoder Velocity") -> ("Numeric"=→"Top Encoder Velocity":dbl)  [unwired: 9 in, 1 out]
        n110 = call-poly <vilib>:"NT Write Value.vi"("Boolean"="PID Control", "Name"="PID Control") -> ()  [unwired: 9 in, 1 out]
        n111 = call "Prepare Joystick Data for Displays.vi"("Joystick Values"=w238) -> ("Buttons"=→"JS2 Buttons":T21, "Z Axis"=→"JS2 Z":dbl, "Cartesian Data"=→"JS2 Graph":cluster{"X axis":dbl, "X axis":dbl}[])  [unwired: 8 in]
        n112 = call "Prepare Joystick Data for Displays.vi"("Joystick Values"=w243) -> ("Buttons"=→"JS1 Buttons":T21, "Z Axis"=→"JS1 Z":dbl, "Cartesian Data"=→"JS1 Graph":cluster{"X axis":dbl, "X axis":dbl}[])  [unwired: 8 in]
        n113 = Bundle("Numeric"=w246, "Numeric"=w247) -> ()  [unwired: 1 in, 1 out]
        n114 = Bundle("Numeric"=w248, "Numeric"=w251, "Battery V"=w245) -> ()  [unwired: 1 in, 1 out]
        n115 = call-poly <vilib>:"NT Read Value.vi"("Name"="Top Limit") -> ("Boolean"=→"Top Wop":bool)  [unwired: 9 in, 1 out]
        n116 = call-poly <vilib>:"NT Write Value.vi"("Numeric"="Top Speed", "Name"="Top Speed") -> ()  [unwired: 9 in, 1 out]
        n117 = call-poly <vilib>:"NT Write Value.vi"("Numeric"="Bottom Speed", "Name"="Bottom Speed") -> ()  [unwired: 9 in, 1 out]
        n118 = call-poly <vilib>:"NT Read Value.vi"("Name"="Bottom Limit") -> ("Boolean"=→"Bottom Floop":bool)  [unwired: 9 in, 1 out]
        n119 = call-poly <vilib>:"NT Write Value.vi"("Numeric"="Intake Speed", "Name"="Intake Speed") -> ()  [unwired: 9 in, 1 out]
        n120 = disable-structure shown="Disabled" {
          frame Disabled {
            n121 = call-poly <vilib>:"SD Write Value.vi"("Name"="Top Speed") -> ("Numeric"=w260:dbl)  [unwired: 8 in, 2 out]
            n122 = call-poly <vilib>:"SD Write Value.vi"("Name"="Intake Speed") -> ("Numeric"=w256:dbl)  [unwired: 8 in, 2 out]
            n123 = call-poly <vilib>:"SD Write Value.vi"("Name"="Back Speed") -> ("Numeric"=w258:dbl)  [unwired: 8 in, 2 out]
          }
          frame Enabled {
          }
        }
        n124 = call-poly <vilib>:"NT Read Value.vi"("Name"="Right Drive Motor") -> ("Numeric"=→"Right Drive Encoder":dbl)  [unwired: 9 in, 1 out]
        n125 = call-poly <vilib>:"NT Read Value.vi"("Name"="Left Drive Motor") -> ("Numeric"=→"Left Drive Encoder":dbl)  [unwired: 9 in, 1 out]
        n126 = call-poly <vilib>:"NT Write Value.vi"("Numeric"="Second Turn", "Name"="Second Turn") -> ()  [unwired: 9 in, 1 out]
        n127 = call-poly <vilib>:"NT Write Value.vi"("Numeric"="Second Drive", "Name"="Second Drive") -> ()  [unwired: 9 in, 1 out]
        n128 = call-poly <vilib>:"NT Read Value.vi"("Name"="Override") -> ("Boolean"=→"Override":bool)  [unwired: 9 in, 1 out]
        n129 = call-poly <vilib>:"NT Write Value.vi"("Numeric"="X Offset", "Name"="X Offset") -> ()  [unwired: 9 in, 1 out]
        n130 = call-poly <vilib>:"NT Write Value.vi"("Numeric"="Top P", "Name"="Top P") -> ()  [unwired: 9 in, 1 out]
        n131 = call-poly <vilib>:"NT Write Value.vi"("Numeric"="Angle Offset", "Name"="Angle Offset") -> ()  [unwired: 9 in, 1 out]
        n132 = call-poly <vilib>:"NT Write Value.vi"("Numeric"="Top D", "Name"="Top D") -> ()  [unwired: 9 in, 1 out]
        n133 = call-poly <vilib>:"NT Write Value.vi"("Numeric"="Top I", "Name"="Top I") -> ()  [unwired: 9 in, 1 out]
        n134 = call-poly <vilib>:"NT Write Value.vi"("Boolean"="Auto Shoot", "Name"="Auto Shoot") -> ()  [unwired: 9 in, 1 out]
        n135 = call-poly <vilib>:"NT Write Value.vi"("Numeric"="First  Drive", "Name"="First Drive") -> ()  [unwired: 9 in, 1 out]
        n136 = call-poly <vilib>:"NT Write Value.vi"("Numeric"="First Turn", "Name"="First Turn") -> ()  [unwired: 9 in, 1 out]
        n137 = call-poly <vilib>:"NT Write Value.vi"("Numeric"="Y Offset", "Name"="Y Offset") -> ()  [unwired: 9 in, 1 out]
        n138 = call-poly <vilib>:"NT Read Value.vi"("Name"="Line Break") -> ("Boolean"=w179:bool)  [unwired: 9 in, 1 out]
        n139 = call-poly <vilib>:"NT Write Value.vi"("Numeric"="Release Speed", "Name"="Release Speed") -> ()  [unwired: 9 in, 1 out]
        n140 = call-poly <vilib>:"NT Write Value.vi"("Numeric"="Bottom P", "Name"="Bottom P") -> ()  [unwired: 9 in, 1 out]
        n141 = call-poly <vilib>:"NT Write Value.vi"("Numeric"="Scale Offset", "Name"="Scale Offset") -> ()  [unwired: 9 in, 1 out]
        n142 = call-poly <vilib>:"NT Write Value.vi"("Numeric"="Bottom D", "Name"="Bottom D") -> ()  [unwired: 9 in, 1 out]
        n143 = Not(x=w179) -> (.not. x?=→"Line  Break":bool)
        n144 = call-poly <vilib>:"NT Write Value.vi"("Numeric"="Bottom I", "Name"="Bottom I") -> ()  [unwired: 9 in, 1 out]
        n145 = call-poly <vilib>:"NT Write Value.vi"("Numeric"="Release Time", "Name"="Release Time") -> ()  [unwired: 9 in, 1 out]
      }
    }
  }
  n146 = property on="Camera Settings" class="Clust (strict)"("Val(Sgnl)"=w55) -> ()  [unwired: 2 in, 2 out]
  n147 = Index Array(array=w52) -> (element=w50:refnum<vi>)  [unwired: 1 in]
  n148 = control-ref of="Test Tree"() -> (w53:refnum<vi>)
  n149 = while {
    tunnel: w56 -> [w279]
    shift-right: [w278] -> _
    shift-left: w54 -> [w277]
    tunnel: [w276] -> _
    tunnel: w53 -> [w275]
    tunnel: w49 -> [w274]
    tunnel: w48 -> [w273]
    tunnel: w47 -> [_]
    tunnel: w43 -> [w272]
    tunnel: w6 -> [w271]
    tunnel: w4 -> [w270]
    shift-right: [w269] -> _
    shift-left: _ -> [w268]
    i -> [w276]
    stop <- FALSE stop-if-true
    n150 = event shown="[0] Timeout" {
      selector: w273 -> [_ _ _ _ _ _ _ _ _ _ _ _ _ _ _ _ _ _ _ _ _ _ _ _]
      dyn-events: [_ _ _ _ _ _ _ _ _ _ _ _ _ _ _ _ _ _ w587 _ _ _ _ _] -> _
      timeout: u32 60 ("milliseconds to wait") -> [_ _ _ _ _ _ _ _ _ _ _ _ _ _ _ _ _ _ _ _ _ _ _ _]
      tunnel: w275 -> [w291 _ _ _ _ _ _ _ _ _ _ _ _ _ _ _ _ _ _ _ _ _ _ _]
      tunnel: "Test Tree" -> [_ _ _ _ _ _ _ _ _ _ _ _ _ w550 w559 w562 w567 w576 _ _ _ _ _ _]
      tunnel: w279 -> [_ w329 _ _ _ _ _ _ _ _ _ w512 w543 _ _ _ _ _ _ _ _ _ _ _]
      tunnel: [w288 w328 w432 w438 w448 w452 w458 w470 w478 w484 w497 w511 w536 w549 w557 w561 w566 w575 w589 w605 w607 w615 w626 w631] -> w278
      tunnel: w277 -> [w288 w328 w432 w438 w448 w452 w458 w470 w478 w484 w497 w510 w536 w549 w557 w561 w566 w575 w589 w605 w607 w615 w626 w631]
      tunnel: w274 -> [_ _ _ _ _ _ _ _ _ _ _ _ _ _ _ _ _ _ w590 _ w610 _ _ _]
      tunnel: w272 -> [_ _ _ _ _ _ _ _ _ _ _ _ _ _ _ _ _ _ w585 _ _ _ _ _]
      tunnel: w271 -> [_ _ _ _ _ _ _ _ _ _ _ _ _ _ _ _ _ _ w581 _ _ _ _ _]
      tunnel: w270 -> [w284 _ _ _ _ _ w456 _ _ _ _ _ _ _ _ _ _ _ _ _ _ _ _ _]
      tunnel: [w283 w327 w431 w437 w447 w453 w454 w464 w475 w483 w496 w509 w535 w548 w556 w560 w565 w574 w580 w603 w606 w611 w619 w632] -> w269
      tunnel: w268 -> [w283 w327 w431 w437 w447 w453 w454 _ _ w483 w496 w509 w535 w548 w556 w560 w565 w574 w580 w603 w606 w611 w619 w632]
      event Timeout {
        n151 = event-data() -> ()  [unwired: 1 in, 1 out]
        n152 = local read "Mode"() -> (w286:T4)
        n153 = call <vilib>:"NT Read String.vi"("Name"="/TestMode/TestName") -> ("String"=w294:string)  [unwired: 9 in, 1 out]
        n154 = case shown="\"Variables\"" "Dashboard Tab" {
          tunnel: w291 -> [_ w305 _ _]
          tunnel: "/TestMode/Automatic/" ("Name Pattern") -> [_ w304 _ _]
          tunnel: T22 [{"Operation"=enum."Clear", "Color Box"=14013909}, {"Operation"=enum."Clear", "Color Box"=14013909}, {"Operation"=enum."Clear", "Color Box"=14013909}, {"Operation"=enum."Clear", "Color Box"=14013909}, {"Operation"=enum."Update", "Color Box"=14013909}, {"Operation"=enum."Update", "Color Box"=16777215}, {"Operation"=enum."Clear", "Color Box"=14013909}, {"Operation"=enum."Clear", "Color Box"=14013909}, {"Operation"=enum."Clear", "Color Box"=14013909}] -> [_ w297 _ w314]
          tunnel: w286 -> [_ w296 _ w313]
          tunnel: u32[] [15790320, 15790320, 15790320, 15790320, 16777215, 16777215, 15790320, 15790320, 15790320] -> [_ _ _ w319]
          tunnel: w284 -> [_ _ _ w307]
          frame "Custom", Default {
          }
          frame "Test" {
            w303 = -2 ("Active Item:Row Number")
            n155 = Index Array(array=w297, index=w296) -> (element=w298:T26)
            n156 = Unbundle(w298) -> ("Operation"=w299:enum16{"Update", "Clear"}, "Color Box"=w300:u32)
            n157 = call <vilib>:"NT Read and Format Entries as Tree.vi"("Operation"=w299, "Name Pattern"=w304, "Tree Refnum"=w305) -> ()  [unwired: 7 in, 2 out]
            n158 = property on="Test Tree" class="Tree (strict)"("Active Item Row Number"=w303, "ActiveColNum"=w303, "CellBG"=w300, "Active Item Row Number"=-1 ("Active Item:Row Number"), "CellBG"=u32 5789784 ("Color Box")) -> ()  [unwired: 2 in, 2 out]
          }
          frame "Variables" {
            n159 = control-ref of="Tree"() -> (w306:refnum<vi>)
            n160 = call <vilib>:"NT Read and Format Entries as Tree.vi"("Tree Refnum"=w306) -> ()  [unwired: 9 in, 2 out]
          }
          frame "Commands" {
            w315 = u32 5789784 ("Color Box")
            w316 = T27 {"Row"=-1, "Column"=-2} ("Active Cell:Active Cell")
            w318 = T27 {"Row"=-2, "Column"=-2} ("Active Cell:Active Cell")
            n161 = Index Array(array=w319, index=w313) -> (element=w317:u32)
            n162 = Index Array(array=w314, index=w313) -> (element=w312:T26)
            n163 = Unbundle(w312) -> ("Operation"=w311:enum16{"Update", "Clear"})  [unwired: 1 out]
            n164 = local read "Command Selection"() -> (w310:i32)
            n165 = property on="Command Selection" class="MCListbox (strict)"("ActiveCell"=w318, "CellBG"=w317, "ActiveCell"=w316, "CellBG"=w315) -> ()  [unwired: 2 in, 2 out]
            n166 = call <vilib>:"WPI_DashboardUpdate RPC Info.vi"("Operation"=w311) -> ("update"=w309:bool, "commands"=w308:string[][])  [unwired: 9 in]
            n167 = property on="Command Selection" class="MCListbox (strict)"("ItemNames"=w308) -> ()  [unwired: 2 in, 2 out]
            n168 = property on="Command Params" class="Tbl (strict)"("Active Cell"=w318, "Cell BG Color"=w317, "Active Cell"=w316, "Cell BG Color"=w315) -> ()  [unwired: 2 in, 2 out]
            n169 = call <vilib>:"WPI_DashboardUpdate Command Params.vi"("Update"=w309, "NewVal"=w310, "Commands"=w308, "Param Tbl"=w307) -> ()  [unwired: 7 in, 1 out]
          }
        }
        n170 = case shown="Default" w294 {
          tunnel: "/TestMode/TestProgress" ("Name") -> [w321 _]
          tunnel: "/TestMode/TestProgressText" ("Name") -> [w320 _]
          frame Default {
            n171 = call <vilib>:"NT Read Number.vi"("Name"=w321) -> ("Numeric"=w322:dbl)  [unwired: 9 in, 1 out]
            n172 = call <vilib>:"NT Read String.vi"("Name"=w320) -> ("String"=w323:string)  [unwired: 9 in, 1 out]
            n173 = Bundle("Numeric"=w322, "String"=w323) -> (→"Progress":cluster{"Numeric":dbl, "String":string})  [unwired: 1 in]
          }
          frame "" {
            n174 = property on="Progress" class="Clust (strict)"("Visible"=FALSE) -> ()  [unwired: 2 in, 2 out]
            n175 = local write "Test Name"(u16 0) -> ()
          }
        }
        n176 = call <vilib>:"Connextion Info.vi"() -> ()  [unwired: 10 in, 2 out]
      }
      event "Test Tree": Value Change {
        # "Show appropriate\ncontrols"
        n177 = event-data() -> ("CtlRef"=w332:refnum<vi>, "NewVal"=w330:string)  [unwired: 1 in]
        n178 = call <vilib>:"WPI_UtilitiesGetTreeIOName.vi"("NewVal"=w330, "TreeControl in"=w332) -> ("I/O Name"=w333:string)  [unwired: 9 in]
        n179 = case shown="\"Analog Out\", \"Motor\", \"PWM\"" w333 {
          selector: w333 -> [_ w340 _ w362 w371 _]
          tunnel: w330 -> [_ _ w359 w361 _ w378]
          tunnel: w329 -> [_ _ _ _ _ w377]
          frame Default {
            w335 = FALSE ("Visible")
            w334 = FALSE ("Visible")
            n180 = property on="Motor" class="Clust (strict)"("Visible"=w334) -> ()  [unwired: 2 in, 2 out]
            n181 = property on="Test Ring" class="Ring (strict)"("Visible"=w334) -> ()  [unwired: 2 in, 2 out]
            n182 = property on="Rev/Fwd" class="Clust (strict)"("Visible"=w335) -> ()  [unwired: 2 in, 2 out]
            n183 = property on="On/Off" class="Bool (strict)"("Visible"=w335) -> ()  [unwired: 2 in, 2 out]
            n184 = property on="Test Slider" class="Slide (strict)"("Visible"=w335) -> ()  [unwired: 2 in, 2 out]
          }
          frame "Analog Out", "Motor", "PWM" {
            w341 = FALSE ("Visible")
            n185 = case shown="\"Analog Out\"" w340 {
              tunnel: [1.0 ("Value") -1.0 ("Value") 0.0 ("Value")] -> w339
              tunnel: [255.0 ("Value") 1.0 ("Value") 5.0 ("Value")] -> w338
              tunnel: [128.0 ("Value") 0.0 ("Value") 0.0 ("Value")] -> w337
              tunnel: [64.0 ("Value") 0.5 ("Value") 1.0 ("Value")] -> w336
              frame "PWM" {
              }
              frame "Motor", Default {
              }
              frame "Analog Out" {
              }
            }
            n186 = property on="Motor" class="Clust (strict)"("Visible"=TRUE) -> ()  [unwired: 2 in, 2 out]
            n187 = property on="Value" class="Slide (strict)"("Value"=w337, "Scale.Minimum"=w339, "Scale.Maximum"=w338, "Scale.Increment"=w336) -> ()  [unwired: 2 in, 2 out]
            n188 = property on="On/Off" class="Bool (strict)"("Visible"=w341) -> ()  [unwired: 2 in, 2 out]
            n189 = property on="Test Slider" class="Slide (strict)"("Visible"=w341) -> ()  [unwired: 2 in, 2 out]
            n190 = property on="Test Ring" class="Ring (strict)"("Visible"=w341) -> ()  [unwired: 2 in, 2 out]
            n191 = property on="Rev/Fwd" class="Clust (strict)"("Visible"=w341) -> ()  [unwired: 2 in, 2 out]
          }
          frame "Servo" {
            w357 = FALSE ("Visible")
            n192 = call <vilib>:"NT Read Number.vi"("Name"=w359) -> ("Numeric"=w358:dbl)  [unwired: 9 in, 1 out]
            n193 = property on="Test Slider" class="Slide (strict)"("Visible"=TRUE, "Scale.Maximum"=170.0 ("Scale.Range:Maximum")) -> ()  [unwired: 2 in, 2 out]
            n194 = local write "Test Slider"(w358) -> ()
            n195 = property on="Motor" class="Clust (strict)"("Visible"=w357) -> ()  [unwired: 2 in, 2 out]
            n196 = property on="Rev/Fwd" class="Clust (strict)"("Visible"=w357) -> ()  [unwired: 2 in, 2 out]
            n197 = property on="On/Off" class="Bool (strict)"("Visible"=w357) -> ()  [unwired: 2 in, 2 out]
            n198 = property on="Test Ring" class="Ring (strict)"("Visible"=w357) -> ()  [unwired: 2 in, 2 out]
          }
          frame "Relay", "Solenoid" {
            w360 = FALSE ("Visible")
            n199 = property on="Motor" class="Clust (strict)"("Visible"=w360) -> ()  [unwired: 2 in, 2 out]
            n200 = property on="Test Slider" class="Slide (strict)"("Visible"=w360) -> ()  [unwired: 2 in, 2 out]
            n201 = Search and Replace String(input string=w361, search string="/Value  **", replace string="/Direction") -> (result string=w367:string)  [unwired: 5 in, 3 out]
            n202 = property on="Test Ring" class="Ring (strict)"("Visible"=w360) -> ()  [unwired: 2 in, 2 out]
            n203 = call <vilib>:"NT Read String.vi"("Name"=w367) -> ("String"=w365:string)  [unwired: 9 in, 1 out]
            n204 = Equal?(x="Both directions", y=w365) -> (x = y?=w363:bool)
            n205 = Not(x=w363) -> (.not. x?=w364:bool)
            n206 = property on="Rev/Fwd" class="Clust (strict)"("Visible"=w363) -> ()  [unwired: 2 in, 2 out]
            n207 = property on="On/Off" class="Bool (strict)"("Visible"=w364, "Caption.Text"=w362) -> ()  [unwired: 2 in, 2 out]
          }
          frame "Compressor", "Digital Out" {
            w370 = FALSE ("Visible")
            # "Get direction and finish"
            n208 = property on="Motor" class="Clust (strict)"("Visible"=w370) -> ()  [unwired: 2 in, 2 out]
            n209 = property on="Test Slider" class="Slide (strict)"("Visible"=w370) -> ()  [unwired: 2 in, 2 out]
            n210 = property on="Test Ring" class="Ring (strict)"("Visible"=w370) -> ()  [unwired: 2 in, 2 out]
            n211 = property on="On/Off" class="Bool (strict)"("Visible"=TRUE, "Caption.Text"=w371) -> ()  [unwired: 2 in, 2 out]
            n212 = property on="Rev/Fwd" class="Clust (strict)"("Visible"=FALSE) -> ()  [unwired: 2 in, 2 out]
          }
          frame "Camera" {
            n213 = call <vilib>:"Get Last Path Segment.vi"("String in"=w378) -> ("String out"=w379:string)  [unwired: 10 in]
            n214 = property on="On/Off" class="Bool (strict)"("Visible"=FALSE) -> ()  [unwired: 2 in, 2 out]
            n215 = property on="Motor" class="Clust (strict)"("Visible"=FALSE) -> ()  [unwired: 2 in, 2 out]
            n216 = property on="Rev/Fwd" class="Clust (strict)"("Visible"=FALSE) -> ()  [unwired: 2 in, 2 out]
            n217 = case shown="\"White Balance  **\"" w379 {
              tunnel: w378 -> [w385 w394 w403 w412 w421 _ w427]
              tunnel: w377 -> [w383 w391 w400 w409 w418 _ _]
              frame "Size  **" {
                n218 = Index Array(array=w383) -> (element=w382:cluster{string[]})  [unwired: 1 in]
                n219 = call <vilib>:"NT Read String.vi"("Name"=w385) -> ("String"=w384:string)  [unwired: 9 in, 1 out]
                n220 = Unbundle(w382) -> (w380:string[])
                n221 = Match First String(2:w380, 3:w384) -> (0:w381:i32)  [unwired: 1 out]
                n222 = property on="Test Ring" class="Ring (strict)"("Value"=w381, "Strings []"=w380) -> ()  [unwired: 2 in, 2 out]
                n223 = property on="Test Ring" class="Ring (strict)"("Visible"=TRUE) -> ()  [unwired: 2 in, 2 out]
                n224 = property on="Test Slider" class="Slide (strict)"("Visible"=FALSE) -> ()  [unwired: 2 in, 2 out]
              }
              frame "White Balance  **" {
                n225 = Index Array(array=w391, index=1) -> (element=w392:cluster{string[]})
                n226 = call <vilib>:"NT Read String.vi"("Name"=w394) -> ("String"=w393:string)  [unwired: 9 in, 1 out]
                n227 = Unbundle(w392) -> (w389:string[])
                n228 = Match First String(2:w389, 3:w393) -> (0:w388:i32)  [unwired: 1 out]
                n229 = property on="Test Ring" class="Ring (strict)"("Value"=w388, "Strings []"=w389) -> ()  [unwired: 2 in, 2 out]
                n230 = property on="Test Ring" class="Ring (strict)"("Visible"=TRUE) -> ()  [unwired: 2 in, 2 out]
                n231 = property on="Test Slider" class="Slide (strict)"("Visible"=FALSE) -> ()  [unwired: 2 in, 2 out]
              }
              frame "Exposure  **" {
                n232 = Index Array(array=w400, index=2) -> (element=w401:cluster{string[]})
                n233 = call <vilib>:"NT Read String.vi"("Name"=w403) -> ("String"=w402:string)  [unwired: 9 in, 1 out]
                n234 = Unbundle(w401) -> (w397:string[])
                n235 = Match First String(2:w397, 3:w402) -> (0:w398:i32)  [unwired: 1 out]
                n236 = property on="Test Ring" class="Ring (strict)"("Value"=w398, "Strings []"=w397) -> ()  [unwired: 2 in, 2 out]
                n237 = property on="Test Ring" class="Ring (strict)"("Visible"=TRUE) -> ()  [unwired: 2 in, 2 out]
                n238 = property on="Test Slider" class="Slide (strict)"("Visible"=FALSE) -> ()  [unwired: 2 in, 2 out]
              }
              frame "Exposure Priority  **" {
                n239 = Index Array(array=w409, index=3) -> (element=w410:cluster{string[]})
                n240 = call <vilib>:"NT Read String.vi"("Name"=w412) -> ("String"=w411:string)  [unwired: 9 in, 1 out]
                n241 = Unbundle(w410) -> (w406:string[])
                n242 = Match First String(2:w406, 3:w411) -> (0:w407:i32)  [unwired: 1 out]
                n243 = property on="Test Ring" class="Ring (strict)"("Value"=w407, "Strings []"=w406) -> ()  [unwired: 2 in, 2 out]
                n244 = property on="Test Ring" class="Ring (strict)"("Visible"=TRUE) -> ()  [unwired: 2 in, 2 out]
                n245 = property on="Test Slider" class="Slide (strict)"("Visible"=FALSE) -> ()  [unwired: 2 in, 2 out]
              }
              frame "Color Enable  **" {
                n246 = Index Array(array=w418, index=4) -> (element=w419:cluster{string[]})
                n247 = call <vilib>:"NT Read String.vi"("Name"=w421) -> ("String"=w420:string)  [unwired: 9 in, 1 out]
                n248 = Unbundle(w419) -> (w415:string[])
                n249 = Match First String(2:w415, 3:w420) -> (0:w416:i32)  [unwired: 1 out]
                n250 = property on="Test Ring" class="Ring (strict)"("Value"=w416, "Strings []"=w415) -> ()  [unwired: 2 in, 2 out]
                n251 = property on="Test Ring" class="Ring (strict)"("Visible"=TRUE) -> ()  [unwired: 2 in, 2 out]
                n252 = property on="Test Slider" class="Slide (strict)"("Visible"=FALSE) -> ()  [unwired: 2 in, 2 out]
              }
              frame Default {
                n253 = property on="Test Ring" class="Ring (strict)"("Visible"=FALSE) -> ()  [unwired: 2 in, 2 out]
                n254 = property on="Test Slider" class="Slide (strict)"("Visible"=FALSE) -> ()  [unwired: 2 in, 2 out]
              }
              frame "Brightness  **", "Color Level  **", "Compression  **", "FPS  **", "Sharpness  **" {
                n255 = call <vilib>:"NT Read Number.vi"("Name"=w427) -> ("Numeric"=w426:dbl)  [unwired: 9 in, 1 out]
                n256 = local write "Test Slider"(w426) -> ()
                n257 = property on="Test Slider" class="Slide (strict)"("Visible"=TRUE, "Scale.Maximum"=100.0 ("Scale.Range:Maximum")) -> ()  [unwired: 2 in, 2 out]
                n258 = property on="Test Ring" class="Ring (strict)"("Visible"=FALSE) -> ()  [unwired: 2 in, 2 out]
              }
            }
          }
        }
        n259 = property on="Progress" class="Clust (strict)"("Visible"=FALSE) -> ()  [unwired: 2 in, 2 out]
      }
      event "Test Name": Mouse Enter {
        # "Populate the ring with the list of tests"
        n260 = event-data() -> ()  [unwired: 1 in, 1 out]
        n261 = call <vilib>:"NT Read String Array.vi"("Name"="/TestMode/TestList") -> ("String Array"=w436:string[])  [unwired: 9 in, 1 out]
        n262 = Build Array (concatenate)("Select the test to run...", w436) -> (w435:string[])
        n263 = property on="Test Name" class="Ring (strict)"("Strings []"=w435) -> ()  [unwired: 2 in, 2 out]
      }
      event "Test Name": Value Change {
        w439 = FALSE ("Visible")
        # "Tell the robot the test name to run"
        n264 = event-data() -> ("NewVal"=w443:u16)  [unwired: 1 in]
        n265 = property on="Test Name" class="Ring (strict)"() -> ("Strings []"=w444:string[])  [unwired: 2 in, 2 out]
        n266 = local write "Progress"(T6 {"Test Progress"=0, "Test Progress Text"=""} ("Progress")) -> ()
        n267 = Index Array(array=w444, index=w443) -> (element=w442:string)
        n268 = call <vilib>:"NT Write String.vi"("String"=w442, "Name"="/TestMode/TestName") -> ()  [unwired: 9 in, 1 out]
        n269 = property on="Progress" class="Clust (strict)"("Visible"=TRUE) -> ()  [unwired: 2 in, 2 out]
        n270 = property on="Motor" class="Clust (strict)"("Visible"=w439) -> ()  [unwired: 2 in, 2 out]
        n271 = property on="Test Slider" class="Slide (strict)"("Visible"=w439) -> ()  [unwired: 2 in, 2 out]
        n272 = property on="On/Off" class="Bool (strict)"("Visible"=w439) -> ()  [unwired: 2 in, 2 out]
        n273 = property on="Rev/Fwd" class="Clust (strict)"("Visible"=w439) -> ()  [unwired: 2 in, 2 out]
        n274 = property on="Test Ring" class="Ring (strict)"("Visible"=w439) -> ()  [unwired: 2 in, 2 out]
      }
      event "Select Auto": Mouse Enter {
        # "Populate the combo box with the list of autonomous options"
        n275 = event-data() -> ()  [unwired: 1 in, 1 out]
        n276 = call <vilib>:"NT Read String Array.vi"("Name"="Auto List") -> ("String Array"=w446:string[])  [unwired: 9 in, 1 out]
        n277 = property on="Select Auto" class="CmbBox"("Strings[]"=w446) -> ()  [unwired: 2 in, 2 out]
      }
      event "Select Auto": Value Change {
        # "User modified the Auto Selection. Write to NT variable so robot knows."
        n278 = event-data() -> ("NewVal"=w450:string)  [unwired: 1 in]
        n279 = call <vilib>:"NT Write String.vi"("String"=w450, "Name"="Auto Selector") -> ()  [unwired: 9 in, 1 out]
      }
      event "Command Selection": Value Change {
        # "Get the params and show in table"
        n280 = event-data() -> ("NewVal"=w457:i32)  [unwired: 1 in]
        n281 = property on="Command Selection" class="MCListbox (strict)"() -> ("ItemNames"=w455:string[][])  [unwired: 2 in, 2 out]
        n282 = call <vilib>:"WPI_DashboardUpdate Command Params.vi"("NewVal"=w457, "Commands"=w455, "Param Tbl"=w456) -> ()  [unwired: 8 in, 1 out]
      }
      event "Execute Command": Value Change {
        # "Started one, Unique ID holds\nresponse"
        n283 = event-data() -> ()  [unwired: 1 in, 1 out]
        n284 = property on="Command Selection" class="MCListbox (strict)"() -> ("ItemNames"=w469:string[][])  [unwired: 2 in, 2 out]
        n285 = Index Array(array=w469, index (row)="Command Selection", index (col)=0) -> (element=w467:string)
        n286 = call <vilib>:"Invoke Commands.vi"("Command Params"="Command Params", "Function Name"=w467) -> ("Params"=w463:u8, "Started"=w462:bool)  [unwired: 7 in, 1 out]
        n287 = Array Subset(array="Command Params", length (row)=w463) -> (w464:string[][])  [unwired: 3 in]
        n288 = Select(t="Executing" ("Cmd Status"), s=w462, f="" ("Cmd Status")) -> (s? t:f=→"Cmd Status":string)
      }
      event "Command Selection": Double Click {
        n289 = event-data() -> ("Row"=w479:i32)  [unwired: 1 in]
        n290 = property on="Command Selection" class="MCListbox (strict)"() -> ("ItemNames"=w482:string[][])  [unwired: 2 in, 2 out]
        n291 = local read "Command Params"() -> (w477:string[][])
        n292 = Index Array(array=w482, index (row)=w479, index (col)=0) -> (element=w480:string)
        n293 = call <vilib>:"Invoke Commands.vi"("Command Params"=w477, "Function Name"=w480) -> ("Params"=w476:u8, "Started"=w471:bool)  [unwired: 7 in, 1 out]
        n294 = Array Subset(array=w477, length (row)=w476) -> (w475:string[][])  [unwired: 3 in]
        n295 = Select(t="Executing" ("Cmd Status"), s=w471, f="" ("Cmd Status")) -> (s? t:f=w472:string)
        n296 = local write "Cmd Status"(w472) -> ()
      }
      event "CheckList": Double Click {
        # "Shift clears all"
        # "Update symbols on the listbox"
        n297 = event-data() -> ("PlatMods.Shift"=w485:bool, "Row"=w487:i32)  [unwired: 1 in]
        n298 = case shown="True" w485 {
          tunnel: w487 -> [w491 _]
          tunnel: 1 -> [w490 _]
          frame False {
            n299 = property on="CheckList" class="LstBox (strict)"() -> ("Item Symbols"=w489:i32[])  [unwired: 2 in, 2 out]
            n300 = Replace Array Subset(array=w489, new element=w490, index=w491) -> (w488:i32[])
            n301 = property on="CheckList" class="LstBox (strict)"("Item Symbols"=w488) -> ()  [unwired: 2 in, 2 out]
          }
          frame True {
            w492 = 0 ("Top Row")
            n302 = property on="CheckList" class="LstBox (strict)"() -> ("Number of Rows"=w494:u32)  [unwired: 2 in, 2 out]
            n303 = Initialize Array(0, w494) -> (w493:i32[])
            n304 = property on="CheckList" class="LstBox (strict)"("Top Row"=w492, "Value"=w492, "Item Symbols"=w493) -> ()  [unwired: 2 in, 2 out]
          }
        }
      }
      event "CheckList": Key Down {
        # "Update symbols on the listbox\nLeft and right keys check and uncheck"
        n305 = event-data() -> ("VKey"=w499:T23)  [unwired: 1 in]
        n306 = case shown="\"Left\", \"Right\"" w499 {
          selector: w499 -> [w504 _]
          tunnel: eventvkey."Left" ("VKey") -> [w502 _]
          frame "Left", "Right" {
            n307 = Equal?(x=w502, y=w504) -> (x = y?=w503:bool)
            n308 = Select(t=0, s=w503, f=1) -> (s? t:f=w505:i32)
            n309 = property on="CheckList" class="LstBox (strict)"() -> ("Item Symbols"=w508:i32[])  [unwired: 2 in, 2 out]
            n310 = Replace Array Subset(array=w508, new element=w505, index="CheckList") -> (w507:i32[])
            n311 = property on="CheckList" class="LstBox (strict)"("Item Symbols"=w507) -> ()  [unwired: 2 in, 2 out]
          }
          frame Default {
          }
        }
      }
      event "DB Camera Config": Value Change {
        # "Show or hide the cluster of controls, store in ini file"
        n312 = event-data() -> ("NewVal"=w513:bool)  [unwired: 1 in]
        n313 = case shown="False" w513 {
          tunnel: w512 -> [w522 _]
          tunnel: [w515 w533] -> w511
          tunnel: w510 -> [w514 w533]
          frame False {
            w529 = "Camera"
            w532 = FALSE ("Visible")
            n314 = local read "Camera Settings"() -> (w521:T3)
            n315 = Index Array(array=w522) -> (element=w525:cluster{string[]})  [unwired: 1 in]
            n316 = Unbundle(w521) -> ("Frame Rate"=w520:i32, "Compression"=w519:i32, "Size"=w523:u16)
            n317 = Unbundle(w525) -> (w524:string[])
            n318 = Index Array(array=w524, index=w523) -> (element=w518:string)
            n319 = call-poly <vilib>:"Write Key.vi"("section"=w529, "value"=w518, "key"="Size", "refnum"=w514) -> ("refnum out"=w531:T14)  [unwired: 2 in, 5 out]
            n320 = call-poly <vilib>:"Write Key.vi"("section"=w529, "value"=w520, "key"="FrameRate", "refnum"=w531) -> ("refnum out"=w530:T14)  [unwired: 1 in, 6 out]
            n321 = property on="Camera Settings" class="Clust (strict)"("Visible"=w532) -> ()  [unwired: 2 in, 2 out]
            n322 = local write "DB Camera Config"(w532) -> ()
            n323 = call-poly <vilib>:"Write Key.vi"("section"=w529, "value"=w519, "key"="Compression", "refnum"=w530) -> ("refnum out"=w516:T14)  [unwired: 1 in, 6 out]
            n324 = call <vilib>:"Close Config Data.vi"("refnum"=w516) -> ("file path"=w517:path)  [unwired: 2 in, 8 out]
            n325 = call <vilib>:"Open Config Data.vi"("configuration file path"=w517) -> ("refnum"=w515:T14)  [unwired: 8 in, 2 out]
          }
          frame True {
            n326 = property on="Camera Settings" class="Clust (strict)"("Visible"=TRUE) -> ()  [unwired: 2 in, 2 out]
          }
        }
      }
      event "Camera Settings": Value Change {
        # "Update summary string when any elements of DB camera change"
        n327 = event-data() -> ("NewVal"=w547:T3)  [unwired: 1 in]
        n328 = Index Array(array=w543) -> (element=w542:cluster{string[]})  [unwired: 1 in]
        n329 = Unbundle(w547) -> ("Frame Rate"=w538:i32, "Compression"=w537:i32, "Size"=w540:u16)
        n330 = Unbundle(w542) -> (w541:string[])
        n331 = Index Array(array=w541, index=w540) -> (element=w539:string)
        n332 = Format Into String(format string="%s   %dfps   %d%%", w539, w538, w537) -> (resulting string=w544:string)  [unwired: 2 in, 1 out]
        n333 = Build Array(w544) -> (w545:string[])
        n334 = property on="DB Camera Config" class="Bool (strict)"("Strings [4]"=w545) -> ()  [unwired: 2 in, 2 out]
      }
      event "Motor.Enable": Value Change {
        # "When the test mode otor enable helper is set, update that\ntree row item's value"
        n335 = event-data() -> ("NewVal"=w554:bool)  [unwired: 1 in]
        n336 = Unbundle("Motor") -> ("Value"=w553:dbl)  [unwired: 1 out]
        n337 = Select(t=w553, s=w554, f=0.0) -> (s? t:f=w551:dbl)
        n338 = call <vilib>:"NT Write Number.vi"("Numeric"=w551, "Name"=w550) -> ()  [unwired: 9 in, 1 out]
      }
      event "Test Slider": Value Change {
        # "When the test mode slider helper is set, update that\ntree row item's value"
        n339 = event-data() -> ("NewVal"=w558:dbl)  [unwired: 1 in]
        n340 = call <vilib>:"NT Write Number.vi"("Numeric"=w558, "Name"=w559) -> ()  [unwired: 9 in, 1 out]
      }
      event "On/Off": Value Change {
        # "When the test mode on/off helper value is set, update that\ntree row item's value"
        n341 = event-data() -> ("NewVal"=w564:bool)  [unwired: 1 in]
        n342 = Boolean To (0,1)(Boolean=w564) -> (0, 1=w563:i16)
        n343 = call <vilib>:"NT Write Number.vi"("Numeric"=w563, "Name"=w562) -> ()  [unwired: 9 in, 1 out]
      }
      event "Rev/Fwd": Value Change {
        # "When the test mode helper value for relays is set, update that\ntree row item's value"
        n344 = event-data() -> ("NewVal.Forward"=w573:bool, "NewVal.Reverse"=w572:bool)  [unwired: 1 in]
        n345 = Boolean To (0,1)(Boolean=w573) -> (0, 1=w569:i16)
        n346 = Boolean To (0,1)(Boolean=w572) -> (0, 1=w571:i16)
        n347 = Negate(x=w571) -> (-x=w570:i16)
        n348 = Add(x=w569, y=w570) -> (x+y=w568:i16)
        n349 = call <vilib>:"NT Write Number.vi"("Numeric"=w568, "Name"=w567) -> ()  [unwired: 9 in, 1 out]
      }
      event "Test Ring": Value Change {
        # "When a test mode helper value is selected from the ring,\nset the tree item's variable to the string value"
        n350 = event-data() -> ("NewVal"=w578:u16)  [unwired: 1 in]
        n351 = property on="Test Ring" class="Ring (strict)"() -> ("Strings []"=w579:string[])  [unwired: 2 in, 2 out]
        n352 = Index Array(array=w579, index=w578) -> (element=w577:string)
        n353 = call <vilib>:"NT Write String.vi"("String"=w577, "Name"=w576) -> ()  [unwired: 9 in, 1 out]
      }
      event "Rec Mode": Value Change {
        # "Update globals for recording mode and path to read log from.\nClear when logging and let NetworkTables set path for vision to\nuse."
        n354 = event-data() -> ("NewVal"=w591:enum32{"Stop", "Record", "Playback"})  [unwired: 1 in]
        n355 = global write "WPI_DashboardLogging Global.vi" "Logging Filename"(path "") -> ()
        n356 = global write "WPI_DashboardLogging Global.vi" "Recording"(w591) -> ()
        n357 = case shown="\"Playback\"" w591 {
          tunnel: w590 -> [_ w593 w602]
          tunnel: [_ _ w601] -> w587
          tunnel: [_ _ w600] -> _
          tunnel: w585 -> [_ _ w598]
          tunnel: cluster{i32, i32} {-250, 170} -> [_ _ w597]
          tunnel: [_ _ T24 {"Image Size"=TRUE, "Image Type"=TRUE, "Pixel Value"=TRUE, "ROI Information"=TRUE, "Zoom Factor"=FALSE} ("Image Information Shown:All Elements")] -> w583
          tunnel: [_ _ TRUE ("Zoom Factor")] -> w582
          tunnel: w581 -> [_ _ w594]
          frame Default {
          }
          frame "Stop", "Record" {
            # "Place Window too"
            n358 = invoke class="VI" method="FP.Close"(reference=w593) -> (reference out=w592:refnum<vi>)  [unwired: 2 in, 2 out]
            n359 = invoke class="VI" method="Abort VI"(reference=w592) -> ()  [unwired: 2 in, 3 out]
          }
          frame "Playback" {
            n360 = call "Open Playback Panel.vi"("Offset"=w597, "DB VI Ref"=w598, "Playback in"=w602) -> ("Playback out"=w599:refnum<vi>)  [unwired: 8 in]
            n361 = register-events(w599, w594) -> (reference out=w601:refnum<event-registration>, error out=w600:errorcluster)  [unwired: 2 in]
          }
        }
        n362 = property on="Camera Image" class="ImageControl"("Image Information Shown"=w583, "Image Information Visible"=w582) -> ()  [unwired: 2 in, 2 out]
        n363 = call <vilib>:"WPI_DashboardNT Log FieldName Cache.vi"("Operation"=enum16{"Lookup/Add", "Index", "Clear"}."Clear") -> ()  [unwired: 8 in, 3 out]
      }
      event Panel Close {
        w604 = enum32{"Stop", "Record", "Playback"}."Stop" ("Rec Mode")
        # "Playback window has been closed, abort"
        n364 = event-data() -> ()  [unwired: 1 in, 4 out]
        n365 = local write "Rec Mode"(w604) -> ()
        n366 = global write "WPI_DashboardLogging Global.vi" "Recording"(w604) -> ()
      }
      event Panel Close {
        # "Abort playback window and ourself"
        n367 = event-data() -> ()  [unwired: 1 in, 4 out]
        n368 = invoke class="VI" method="FP.Close"(reference=w610) -> (reference out=w609:refnum<vi>)  [unwired: 2 in, 2 out]
        n369 = invoke class="VI" method="Abort VI"(reference=w609) -> (error out=w608:errorcluster)  [unwired: 2 in, 2 out]
        n370 = invoke class="VI" method="Abort VI"(error in=w608) -> ()  [unwired: 2 in, 3 out]
      }
      event User Event {
        n371 = event-data() -> ("IDs"=w618:cluster{"RPC field ID":u16, "Unique ID":u16}, "String"=w617:string)  [unwired: 1 in]
        n372 = Bundle("IDs"=w618, "String"=w617) -> (w616:T9)  [unwired: 1 in]
        n373 = call <vilib>:"Retrieve RPC Response.vi"("RPC Response"=w616) -> ("Output"=w613:string[][])  [unwired: 10 in]
        n374 = Build Array (concatenate)(w611, w613) -> (w612:string[][])
        n375 = local write "Command Params"(w612) -> ()
        n376 = local write "Cmd Status"("" ("Cmd Status")) -> ()
      }
      event "Vision": Value Change {
        # "Enable/Disable Compression slider.\nHW USB is hard-coded into the camera"
        n377 = event-data() -> ("NewVal"=w625:u16)  [unwired: 1 in]
        n378 = Equal?(x=w625, y=u32 2 ("milliseconds to wait")) -> (x = y?=w623:bool)
        n379 = Select(t=T25."Disabled and Grayed Out" ("Disabled"), s=w623, f=T25."Enabled" ("Disabled")) -> (s? t:f=w620:T25)
        n380 = property on="Compression" class="Slide (strict)"("DisabledEnum"=w620) -> ()  [unwired: 2 in, 2 out]
      }
      event "Tree": Double Click {
        n381 = event-data() -> ("PlatMods"=w630:T28, "Tag"=w629:string)  [unwired: 1 in]
        n382 = Unbundle(w630) -> ("Shift"=w628:bool)  [unwired: 4 out]
        n383 = Not(x=w628) -> (.not. x?=w627:bool)
        n384 = call <vilib>:"NT Update Persistence.vi"("Persistence"=w627, "Name"=w629) -> ()  [unwired: 9 in, 1 out]
      }
    }
  }
  n385 = while {
    tunnel: w50 -> [w634]
    i -> [w637]
    stop <- FALSE stop-if-true
    n386 = Wait (ms)(milliseconds to wait=u32 100) -> ()  [unwired: 1 out]
    n387 = case shown="\"Playback\"" "Rec Mode" {
      tunnel: w637 -> [_ _ w652]
      tunnel: [u32 2829099 ("Base Color") u32 11141120 ("Target Color") w641] -> w633
      frame "Stop", Default {
        # "Reset the color, extra updates don't cost much"
      }
      frame "Record" {
      }
      frame "Playback" {
        # "Playback"
        n388 = Quotient & Remainder(x=w652, y=u32 50 ("milliseconds to wait")) -> (x-y*floor(x/y)=w648:u32)  [unwired: 1 out]
        n389 = Divide(x=w648, y=u32 50 ("milliseconds to wait")) -> (x/y=w645:dbl)
        n390 = Multiply(x=6.283185307179586, y=w645) -> (x*y=w650:dbl)
        n391 = Sine(x=w650) -> (sin(x)=w649:dbl)
        n392 = Absolute Value(x=w649) -> (abs(x)=w642:dbl)
        n393 = call "Interpolate RGB Color.vi"("Proportion"=w642, "Target Color"=u32 30976, "Base Color"=u32 2829099) -> ("Result Color"=w641:u32)  [unwired: 8 in]
      }
    }
    n394 = property class="Pane"(reference=w634, "PaneColor"=w633) -> ()  [unwired: 1 in, 2 out]
  }
  n395 = local write "Dashboard Tab"(T2."Drive" ("Dashboard Tab")) -> ()
  n396 = property on="On/Off" class="Bool (strict)"("Visible"=w18) -> ()  [unwired: 2 in, 2 out]
  n397 = property on="Motor" class="Clust (strict)"("Visible"=w18) -> ()  [unwired: 2 in, 2 out]
  n398 = property on="Progress" class="Clust (strict)"("Visible"=w18) -> ()  [unwired: 2 in, 2 out]
  n399 = property on="Test Ring" class="Ring (strict)"("Visible"=w18) -> ()  [unwired: 2 in, 2 out]
  n400 = property on="Rev/Fwd" class="Clust (strict)"("Visible"=w18) -> ()  [unwired: 2 in, 2 out]
  n401 = property on="Camera Settings" class="Clust (strict)"("Visible"=w18) -> ()  [unwired: 2 in, 2 out]
  n402 = while {
    tunnel: u16 1741 ("timeout ms (25000)") -> [w654]
    stop <- FALSE stop-if-true
    n403 = TCP Create Listener(10:w654) -> (0:w653:errorcluster, 3:w655:refnum<k5>)  [unwired: 4 in, 1 out]
    n404 = case shown="No Error" w653 {
      selector: w653 -> [w657 _]
      tunnel: w655 -> [w658 _]
      frame No Error {
        n405 = while {
          tunnel: w658 -> [w661]
          tunnel: w657 -> [w660]
          stop <- FALSE stop-if-true
          n406 = TCP Wait On Listener(8:w660, 11:w661) -> (0:w662:errorcluster, 4:w663:refnum<k5>)  [unwired: 2 in, 3 out]
          n407 = local write "TCP"(w663) -> ()
          n408 = case shown="No Error" w662 {
            frame No Error {
            }
            frame Error {
              n409 = Wait (ms)(milliseconds to wait=u32 1000) -> ()  [unwired: 1 out]
            }
          }
        }
      }
      frame Error {
        n410 = Wait (ms)(milliseconds to wait=u32 1000) -> ()  [unwired: 1 out]
      }
    }
  }
  n411 = local write "DB Camera Config"(w18) -> ()
  n412 = local write "Command Params"(string[][] [] ("Command Params")) -> ()
  n413 = global write "WPI_DashboardLogging Global.vi" "Recording"(w44) -> ()
  n414 = local write "Command Selection"(u16 0 ("milliseconds to wait")) -> ()
  n415 = local write "Rec Mode"(w44) -> ()
